vi "get_half_display_dim.vi"(8 "Cols":i32, 11 "Rows":i32) -> (0 "Semi Cols":i32, 3 "Semi Rows":i32)   [LabVIEW 2024]
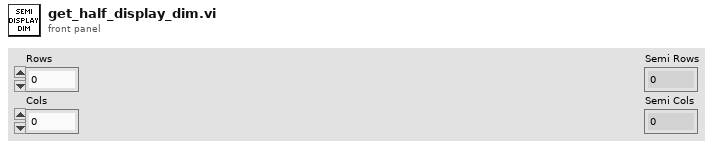
[diagram p1: front panel]
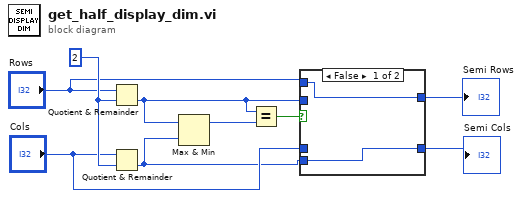
[diagram p0: block diagram]
diagram:
  w9 = 2 ("y")
  n1 = Quotient & Remainder(x="Rows", y=w9) -> (floor(x/y)=w6:i32)  [unwired: 1 out]
  n2 = Quotient & Remainder(x="Cols", y=w9) -> (floor(x/y)=w2:i32)  [unwired: 1 out]
  n3 = Max & Min(x=w6, y=w2) -> (max(x,y)=w8:i32)  [unwired: 1 out]
  n4 = Equal?(x=w6, y=w8) -> (x = y?=w7:bool)
  n5 = case shown="False" w7 {
    tunnel: w6 -> [_ w13]
    tunnel: [w10 w13] -> w5
    tunnel: "Cols" -> [_ w12]
    tunnel: [w11 w12] -> w3
    tunnel: w2 -> [w11 _]
    tunnel: "Rows" -> [w10 _]
    frame False {
    }
    frame True {
    }
  }
  "Semi Rows" <- w5
  "Semi Cols" <- w3
